vi "JSON text to Variant (path).vi"(7 "Item Path":string, 8 "error in (no error)":errorcluster, 9 "Variant (Data Type)":variant, 10 "Starting Offset":i32, 11 "JSON":string) -> (0 "error out":errorcluster, 1 "Variant out":variant, 3 "Found":bool)   [LabVIEW 2017, in "JSONtext.lvlib"]
uses:
  JSONtext.lvlib
  String Subset.vi
  Offset/Find Item Locations by Path.vi
  Parsing/Parse Full Path or Item Name.vi
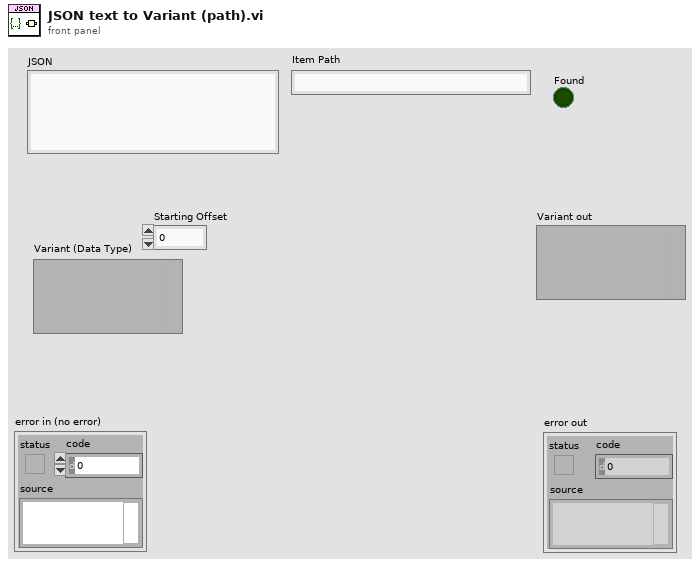
[diagram p1: front panel]
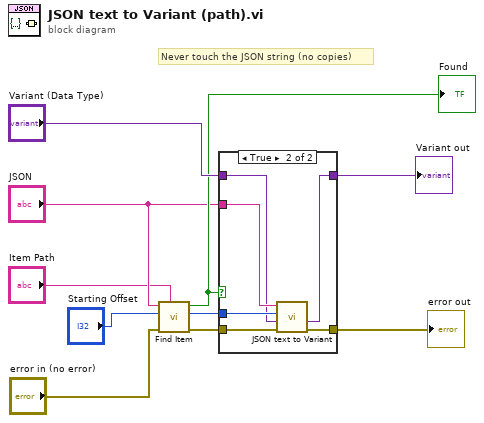
[diagram p0: block diagram]
diagram:
  # "Never touch the JSON string (no copies)"
  n1 = call "Find Item.vi"("$Path or Item Name"="Item Path", "error in (no error)"="error in (no error)", "Offset"="Starting Offset", "JSON"="JSON") -> ("error out"=w8:errorcluster, "Item offset"=w10:i32, "Found"=w4:bool)  [unwired: 4 in, 1 out]
  "Found" <- w4
  n2 = case shown="True" w4 {
    tunnel: "JSON" -> [_ w18]
    tunnel: w10 -> [_ w17]
    tunnel: w8 -> [w11 w16]
    tunnel: "Variant (Data Type)" -> [w12 w15]
    tunnel: [w11 w14] -> w6
    tunnel: [w12 w13] -> w5
    frame False {
    }
    frame True {
      n3 = call "JSON text to Variant.vi"("error in (no error)"=w16, "Data Type"=w15, "Offset"=w17, "JSON"=w18) -> ("error out"=w14:errorcluster, "Variant out"=w13:variant)  [unwired: 6 in]
    }
  }
  "Variant out" <- w5
  "error out" <- w6
